vi "GT Get Thread.vi"(8 "error in (no error)":errorcluster caption="错误输入（无错误）", 9 "pThread":T1, 10 "thread":i16, 11 "cardNum":i16) -> (0 "error out":errorcluster caption="错误输出", 1 "pThread out":T1, 3 "function return":i16)   [LabVIEW 2020, in "gts1.lvlib"]
doc: "GT_API GT_GetThread(short cardNum,short thread,TThreadStatus *pThread);"
uses:
  gts1.lvlib
  dll/32bit/multi_card/gts.dll
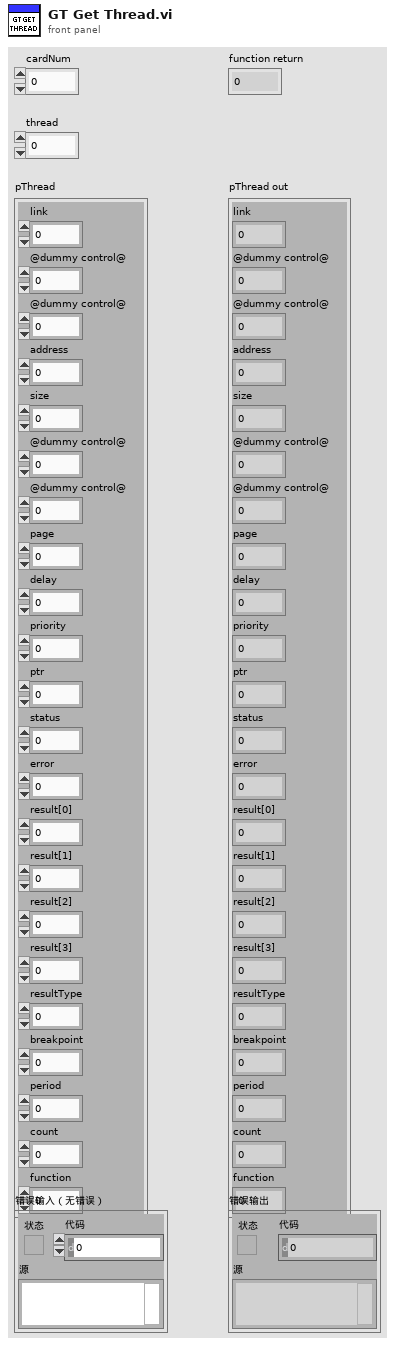
[diagram p1: front panel]
types:
  T1 = cluster{"link":i16, "@dummy control@":i8, "@dummy control@":i8, "address":u32, "size":i16, "@dummy control@":i8, "@dummy control@":i8, "page":u32, "delay":i16, "priority":i16, "ptr":i16, "status":i16, "error":i16, "result[0]":i16, "result[1]":i16, "result[2]":i16, "result[3]":i16, "resultType":i16, "breakpoint":i16, "period":i16, "count":i16, "function":i16}
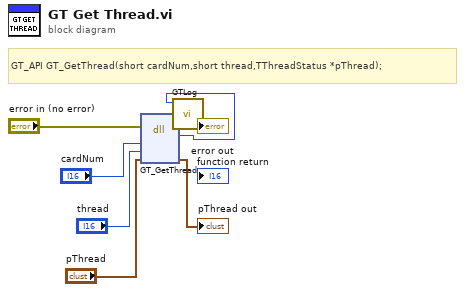
[diagram p0: block diagram]
diagram:
  # "GT_API GT_GetThread(short cardNum,short thread,TThreadStatus *pThread);"
  n1 = dll-call lib="C:/1228/dll/32bit/multi_card/gts.dll" fn="GT_GetThread"(error in="error in (no error)", "cardNum"="cardNum", "thread"="thread", "pThread"="pThread") -> (error out=w3:errorcluster, w1:i16, "pThread"=→"pThread out":T1)  [unwired: 4 in, 1 out]
  n2 = call "GTLog.vi"("error in (no error)"=w3, "Numeric"=w1) -> ("error out"=→"error out":errorcluster)  [unwired: 9 in]
